vi "Check Size Equality.vi"(7 "Command/Response Refnum in":T1 format="%.0x", 8 "Error In":errorcluster, 9 "Variables":string[](array[string]), 11 "Linked Channels in":cluster{"Variable Name":string, "GUID":string}[](array[cluster])) -> (0 "Error Out":errorcluster, 1 "Variables out":string[](array[string]), 3 "Linked Channels out":cluster{"Variable Name":string, "GUID":string}[](array[cluster]))   [LabVIEW 2018, in "Instrument Addon Scripting API.lvlib"]
uses:
  Instrument Addon Scripting API.lvlib
  <vilib>/NI Veristand/Custom Device API/Custom Device Item Ref.ctl
  <vilib>/NI Veristand/Custom Device API/Custom Device API.lvlib
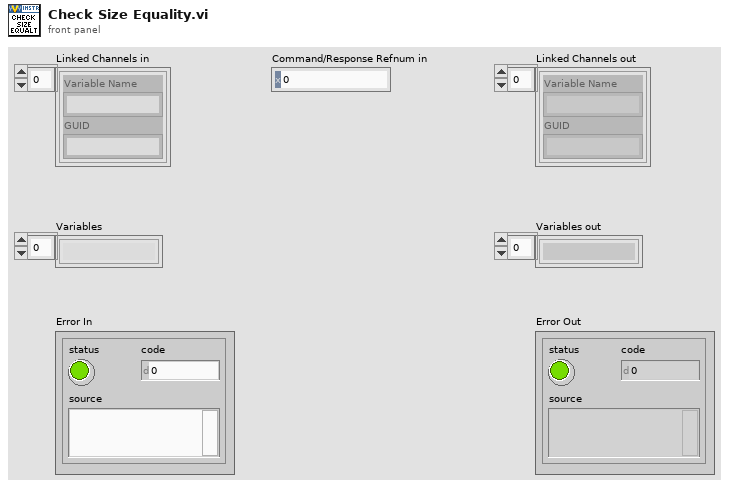
[diagram p1: front panel]
types:
  T1 = typedef "Custom Device API.lvlib/Custom Device Item Ref.ctl" = u64
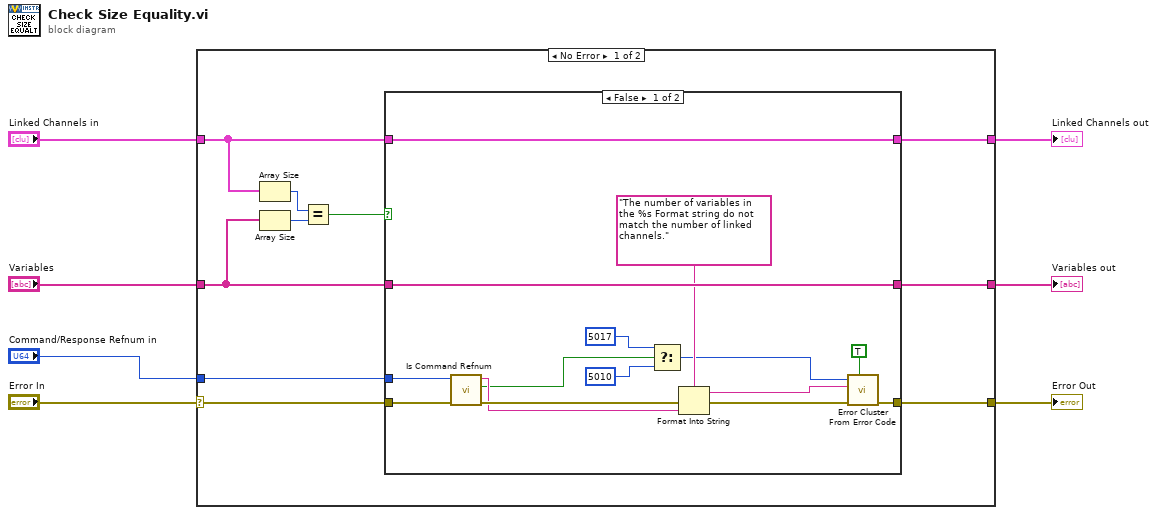
[diagram p0: block diagram]
diagram:
  n1 = case shown="No Error" "Error In" {
    selector: "Error In" -> [w14 w38]
    tunnel: "Variables" -> [w12 w36]
    tunnel: "Linked Channels in" -> [w11 w37]
    tunnel: [w13 w38] -> w4
    tunnel: [w10 w37] -> w3
    tunnel: [w9 w36] -> w2
    tunnel: "Command/Response Refnum in" -> [w8 _]
    frame No Error {
      n2 = Array Size(array=w11) -> (size(s)=w17:i32)
      n3 = Array Size(array=w12) -> (size(s)=w16:i32)
      n4 = Equal?(x=w17, y=w16) -> (x = y?=w15:bool)
      n5 = case shown="False" w15 {
        tunnel: w14 -> [w23 w35]
        tunnel: [w32 w35] -> w13
        tunnel: w12 -> [w30 w33]
        tunnel: w11 -> [w31 w34]
        tunnel: [w31 w34] -> w10
        tunnel: [w30 w33] -> w9
        tunnel: w8 -> [w20 _]
        frame False {
          n6 = call "Is Command Refnum.vi"("error in (no error)"=w23, "Command/Response Refnum in"=w20) -> ("error out"=w22:errorcluster, "Is Command?"=w19:bool, "Command/Response out"=w21:string)  [unwired: 7 in]
          n7 = Select(t=5017 ("error code (0)"), s=w19, f=5010 ("error code (0)")) -> (s? t:f=w24:i32)
          n8 = Format Into String(format string="The number of variables in the %s Format string do not match the number of linked channels." ("error message (\"\")"), error in=w22, w21) -> (resulting string=w27:string, error out=w28:errorcluster)  [unwired: 1 in]
          n9 = call <vilib>:"Error Cluster From Error Code.vi"("show call chain? (False)"=TRUE, "error in (no error)"=w28, "error message (\"\")"=w27, "error code (0)"=w24) -> ("error out"=w32:errorcluster)  [unwired: 5 in]
        }
        frame True {
        }
      }
    }
    frame Error {
    }
  }
  "Error Out" <- w4
  "Linked Channels out" <- w3
  "Variables out" <- w2
